vi "Get total number of commanded axes.vi"(0 "System no.":i32=1 min=1 max=4 step=1, 2 "String":string) -> (14 "Axes":i32, 15 "Equal?":bool, 16 "Commanded Axes":string[](array[string]), 17 "Index of axis":i32[](array[numeric]))   [LabVIEW 2026]
doc: "This VI returns how many axes to command String contains and if that number is equal to the total number of connected axes. Additionally it returns all commanded axes and their index in the Connected Axes array."
panel:
  # "This vi returns how many axes to command String contains and if that number is equal to the total number of \nconnected axes. Additionally it returns all commanded axes and their index in the Connected Axes array."
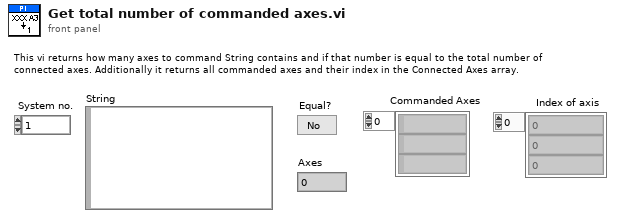
[diagram p1: front panel]
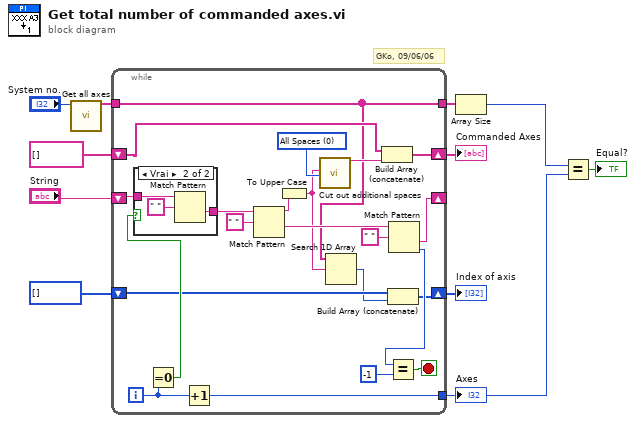
[diagram p0: block diagram]
diagram:
  # "GKo, 09/06/06"
  n1 = call "Get all axes.vi"("System no."="System no.") -> ("Conn. Axes"=w3:string[])  [unwired: 18 out]
  n2 = while {
    shift-right: [w28] -> _
    shift-left: "String" -> [w33]
    tunnel: [w23] -> w8
    shift-right: [w19] -> w5
    shift-left: string[] [] -> [w18]
    tunnel: w3 -> [w16]
    tunnel: [w16] -> w4
    shift-right: [w13] -> w1
    shift-left: i32[] [] -> [w14]
    i -> [w22]
    stop <- w26 stop-if-true
    w20 = u16 0 items=["All Spaces", "Only if 1st char.", "Only if last char.", "Only if near \"=\"", "Only if 1st or last char.", "Only multiple"] ("Mode")
    n3 = Equal To 0?(x=w22) -> (x = 0?=w25:bool)
    n4 = case shown="Vrai" w25 {
      tunnel: w33 -> [w34 w37]
      tunnel: [w34 w35] -> w31
      frame False {
      }
      frame True {
        n5 = Match Pattern(string=w37, regular expression=" ") -> (after substring=w35:string)  [unwired: 4 out]
      }
    }
    n6 = Increment(x=w22) -> (x+1=w23:i32)
    n7 = Match Pattern(string=w31, regular expression=" ") -> (before substring=w21:string, after substring=w29:string)  [unwired: 3 out]
    n8 = To Upper Case(1:w21) -> (0:w15:string)
    n9 = call "Cut out additional spaces.vi"("String"=w15, "Mode"=w20) -> ("String out"=w17:string)  [unwired: 17 out]
    n10 = Search 1D Array(1D array=w16, element=w15) -> (index of element=w12:i32)  [unwired: 1 out]
    n11 = Build Array (concatenate)(w18, w17) -> (w19:string[])
    n12 = Build Array (concatenate)(w14, w12) -> (w13:i32[])
    n13 = Match Pattern(string=w29, regular expression=" ") -> (after substring=w28:string, offset past match=w27:i32)  [unwired: 3 out]
    n14 = Equal?(x=w27, y=-1) -> (x = y?=w26:bool)
  }
  "Axes" <- w8
  "Commanded Axes" <- w5
  "Index of axis" <- w1
  n15 = Array Size(array=w4) -> (size(s)=w9:i32)
  n16 = Equal?(x=w9, y=w8) -> (x = y?=→"Equal?":bool)
